vi "Configure Channel.vi"   [LabVIEW 2022 SP3, in "Agilent U2722.lvlib"]
doc: "Configures the output mode and characteristics of each channel."
uses:
  Agilent U2722.lvlib
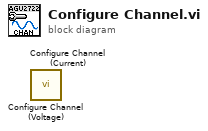
[diagram p0: block diagram]
diagram:
  n1 = call "Configure Channel (Voltage).vi"() -> ()  [unwired: 10 in, 2 out]
  n2 = call "Configure Channel (Current).vi"() -> ()  [unwired: 10 in, 2 out]
